vi "伺服状态.vi"(11 "枚举":enum16{"输入轴驱动", "输入轴移载", "工装移载"}(ring)) -> (3 "Status":sgl)   [LabVIEW 2020]
uses:
  Libraries/S7/S7.lvlib
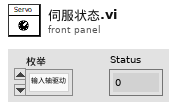
[diagram p1: front panel]
types:
  T1 = typedef "S7.lvlib/Read_Data (Reply Payload)--cluster.ctl" = cluster{"读取成功":bool, "数据":u32[], "Read_Data_error":errorcluster}
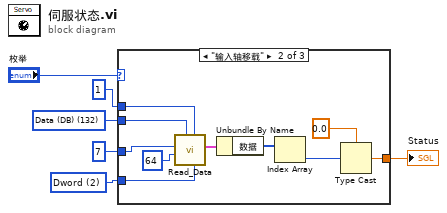
[diagram p0: block diagram]
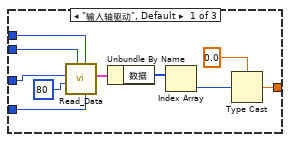
[diagram p2: hidden frame]
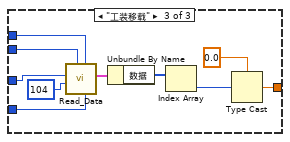
[diagram p3: hidden frame]
diagram:
  w2 = u16 2 items=["byte", "word", "Dword"] ("数据类型")
  w3 = u8 132 items=["I/O (P)"=128, "Input (I)"=129, "Output (Q)"=130, "Bit Memory (M)"=131, "Data (DB)"=132, "Instance Data (DI)"=133, "Local Data (L)"=134, "Predecessor Local Data (VL)"=135] ("寄存器类型")
  n1 = case shown="\"输入轴移载\"" "枚举" {
    tunnel: u16 7 ("DB #") -> [w16 w26 w36]
    tunnel: w3 -> [w12 w22 w32]
    tunnel: u16 1 ("读取长度") -> [w11 w21 w31]
    tunnel: w2 -> [w10 w20 w30]
    tunnel: [w7 w17 w27] -> w1
    frame "输入轴驱动", Default {
      n2 = call "Read_Data.vi"("数据类型"=w10, "读取长度"=w11, "寄存器类型"=w12, "起始地址"=u32 80, "DB #"=w16) -> ("Reply Payload"=w15:T1)  [unwired: 4 in, 2 out]
      n3 = Unbundle By Name(w15) -> ("数据"=w14:u32[])
      n4 = Index Array(array=w14) -> (element=w9:u32)  [unwired: 1 in]
      n5 = Type Cast(type=sgl 0.0, x=w9) -> (*(type *) &x=w7:sgl)
    }
    frame "输入轴移载" {
      n6 = call "Read_Data.vi"("数据类型"=w20, "读取长度"=w21, "寄存器类型"=w22, "起始地址"=u32 64, "DB #"=w26) -> ("Reply Payload"=w25:T1)  [unwired: 4 in, 2 out]
      n7 = Unbundle By Name(w25) -> ("数据"=w24:u32[])
      n8 = Index Array(array=w24) -> (element=w19:u32)  [unwired: 1 in]
      n9 = Type Cast(type=sgl 0.0, x=w19) -> (*(type *) &x=w17:sgl)
    }
    frame "工装移载" {
      n10 = call "Read_Data.vi"("数据类型"=w30, "读取长度"=w31, "寄存器类型"=w32, "起始地址"=u32 104, "DB #"=w36) -> ("Reply Payload"=w35:T1)  [unwired: 4 in, 2 out]
      n11 = Unbundle By Name(w35) -> ("数据"=w34:u32[])
      n12 = Index Array(array=w34) -> (element=w29:u32)  [unwired: 1 in]
      n13 = Type Cast(type=sgl 0.0, x=w29) -> (*(type *) &x=w27:sgl)
    }
  }
  "Status" <- w1
